vi "31_Determinant of 2D array or Matrix.vi"() -> ()   [LabVIEW 2018]
uses:
  <vilib>/Analysis/Matrix/Datatypes/RealMatrix.ctl
  <vilib>/Analysis/baseanly.llb/Real Determinant.vi
  <vilib>/Analysis/NI_AALBase.lvlib
  <vilib>/Analysis/Matrix/NI_Matrix.lvlib
panel:
  out "Determinant":dbl
  in  "Array":dbl[][](array[numeric])
  out "Determinant":dbl
  in  "Real Matrix":T1
  # "Develop a HMI to display determinant of matrix of order 5"
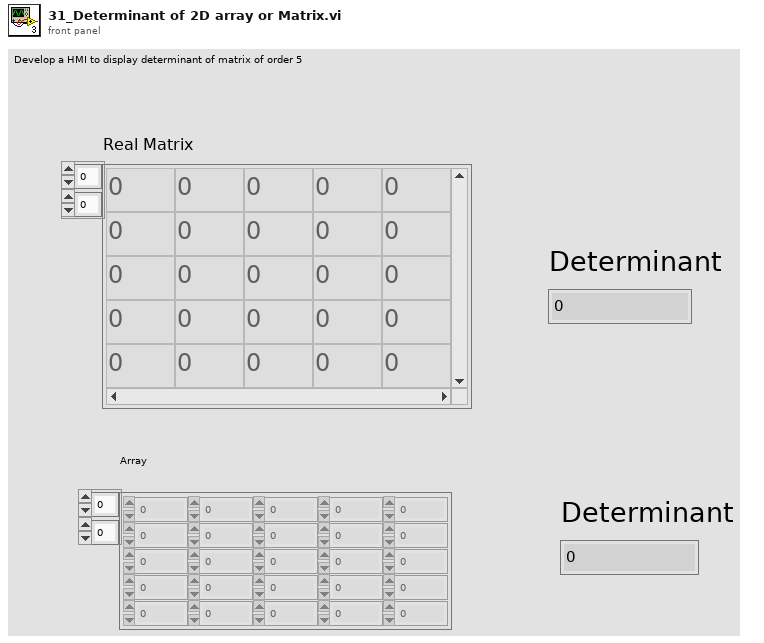
[diagram p1: front panel]
types:
  T1 = typedef "NI_Matrix.lvlib/RealMatrix.ctl" = dbl[][]
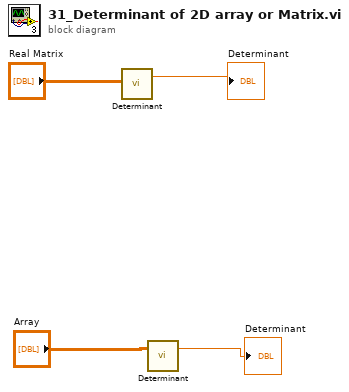
[diagram p0: block diagram]
diagram:
  n1 = call-poly <vilib>:"Determinant.vi"("Input Matrix"="Real Matrix") -> ("determinant"=→"Determinant":dbl)  [unwired: 1 in, 1 out]
  n2 = call-poly <vilib>:"Determinant.vi"("Input Matrix"="Array") -> ("determinant"=→"Determinant":dbl)  [unwired: 1 in, 1 out]
